vi "STARTFIX.vi"() -> ()   [LabVIEW 2024]
uses:
  <vilib>/Utility/file.llb/Read Delimited Spreadsheet (DBL).vi
panel:
  in  "Flow Rate Lower Limit 2":dbl
  in  "Flow Rate Upper Limit 2":dbl
  in  "Desired Flow Rate 3":dbl format="%_2f"
  in  "Initial RPM  3":dbl format="%_4f"
  in  "stop 2":bool
  out "Boolean":bool
  out "Waveform Chart 3":dbl[](graph)
  out "Waveform Chart 2":dbl[](graph)
  out "Flow Rate":dbl(graph)
  in  "Color Box":u32(colorbox)
  # "Blood Flow Rate"
  # "Flow Rate (mL/min)"
  # "Initial LVAD Speed (RPM)"
  # "Desired Flow Rate (mL/min)"
  # "LVAD Speed"
  # "Upper Flow Rate Limit (mL/min)"
  # "Speed (RPM)"
  # "Lower Flow Rate Limit (mL/min)"
  # "Optimal Flow State"
  # "Right Heart Waveform"
  # "Amplitude"
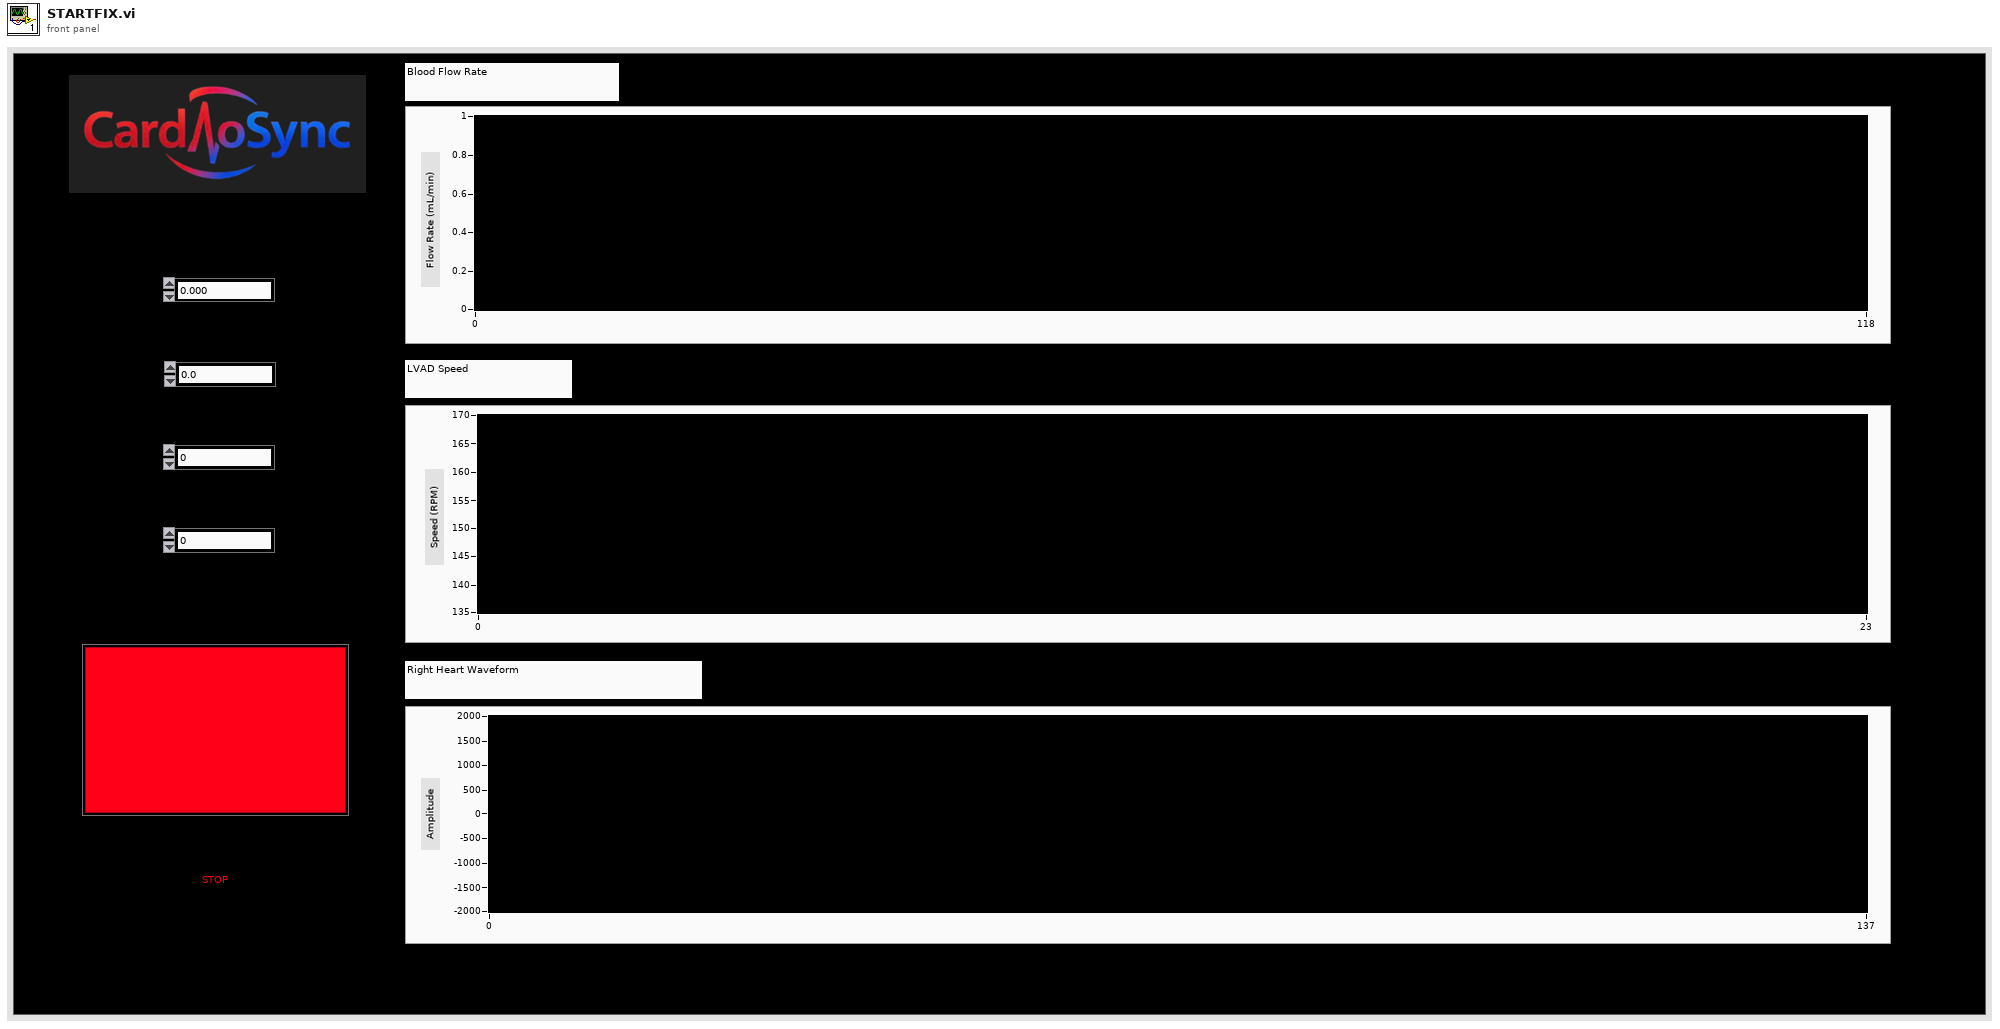
[diagram p1: front panel]
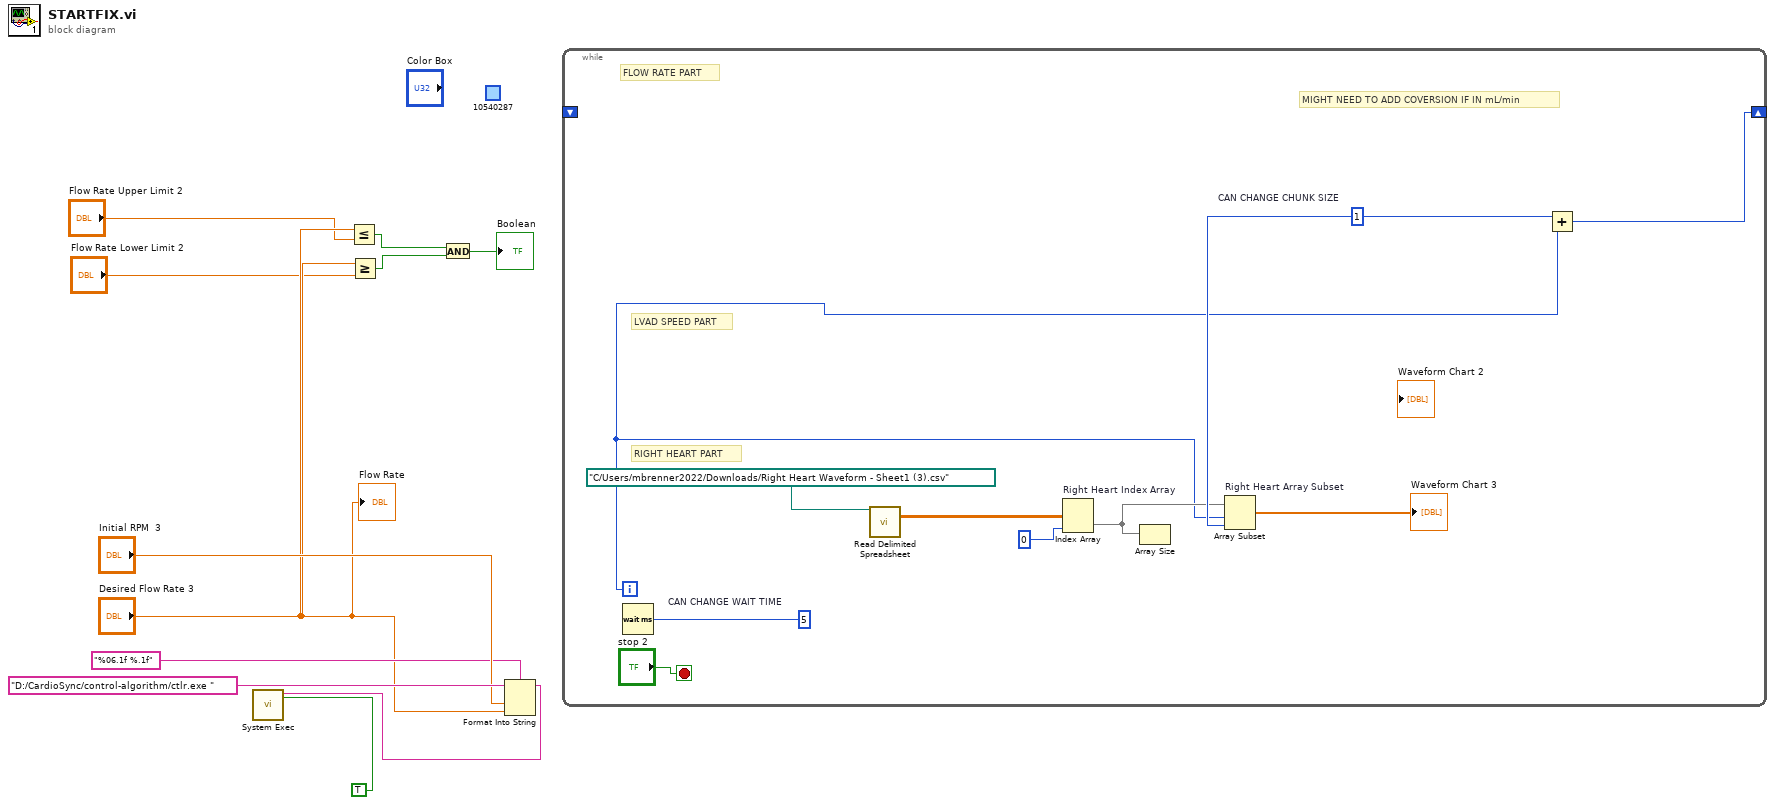
[diagram p0: block diagram]
diagram:
  (unwired) u32 10540287 ("Color Box 2")
  n1 = Less Or Equal?(x="Desired Flow Rate 3", y="Flow Rate Upper Limit 2") -> (x <= y?=w4:bool)
  n2 = Greater Or Equal?(x="Desired Flow Rate 3", y="Flow Rate Lower Limit 2") -> (x >= y?=w5:bool)
  n3 = And(x=w4, y=w5) -> (x .and. y?=→"Boolean":bool)
  n4 = Format Into String(format string="%06.1f %.1f", initial string="D:/CardioSync/control-algorithm/ctlr.exe ", "Initial RPM  3", "Desired Flow Rate 3") -> (resulting string=w8:string)  [unwired: 1 in, 1 out]
  n5 = call <vilib>:"System Exec.vi"("wait until completion? (T)"=TRUE, "command line"=w8) -> ()  [unwired: 6 in, 4 out]
  n6 = while {
    shift-right: [w20] -> _
    shift-left: _ -> [_]
    i -> [w12]
    stop <- "stop 2" stop-if-true
    w21 = u32 5  # CAN CHANGE WAIT TIME
    w17 = 1  # CAN CHANGE CHUNK SIZE
    # "MIGHT NEED TO ADD COVERSION IF IN mL/min"
    # "RIGHT HEART PART"
    # "LVAD SPEED PART"
    # "FLOW RATE PART"
    n7 = Wait (ms)(milliseconds to wait=w21) -> ()  [unwired: 1 out]
    n8 = call-poly <vilib>:"Read Delimited Spreadsheet.vi"("file path (dialog if empty)"=path "C:/Users/mbrenner2022/Downloads/Right Heart Waveform - Sheet1 (3).csv") -> ("all rows"=w18:dbl[][])  [unwired: 9 in, 5 out]
    n9 = Index Array "Right Heart Index Array"(array=w18, index (col)=0 ("disabled index (col)")) -> (element=w14:dbl[])  [unwired: 1 in]
    n10 = Array Size(array=w14) -> ()  [unwired: 1 out]
    n11 = Array Subset "Right Heart Array Subset"(array=w14, index=w12, length=w17) -> (→"Waveform Chart 3":dbl[])
    n12 = Add(x=w17, y=w12) -> (x+y=w20:i32)
  }
  "Flow Rate" <- "Desired Flow Rate 3"
